vi "create_data_file.vi"(7 "Application Directory":string, 8 "Pixel":string, 9 "Device label":string, 10 "Experiment Title":string, 11 "Username":string) -> (2 "Scan number":string, 3 "Filepath out":path)   [LabVIEW 2018]
uses:
  <vilib>/Utility/file.llb/Write Delimited Spreadsheet (string).vi
panel:
  in  "device headings":string[](array[string])=["wavlength (nm)", "current (mA)", "eqe (%)"]
  in  "ref headings":string[](array[string])=["wavelength (nm)", "current (mA)"]
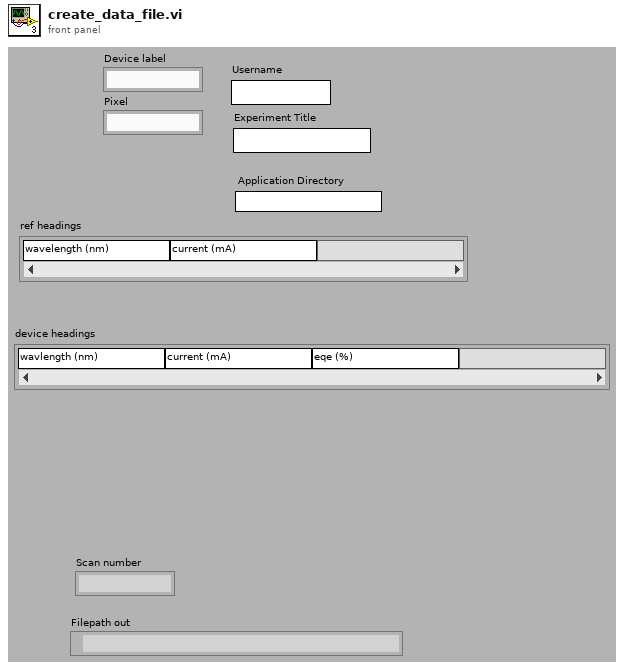
[diagram p1: front panel]
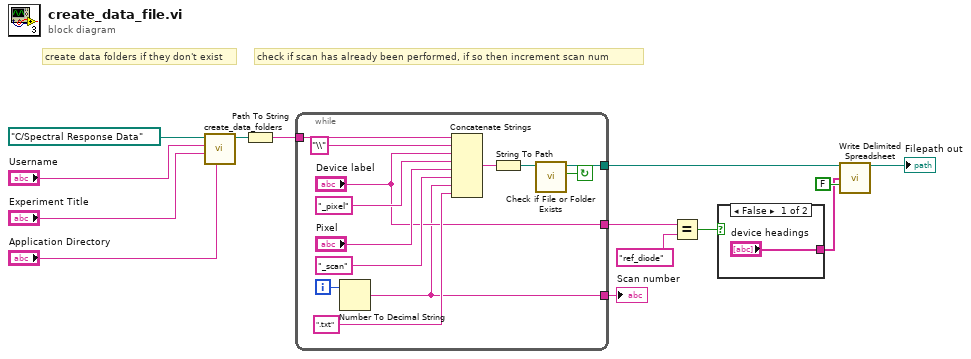
[diagram p0: block diagram]
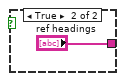
[diagram p2: hidden frame]
diagram:
  # "create data folders if they don't exist"
  # "check if scan has already been performed, if so then increment scan num"
  n1 = call "create_data_folders.vi"("Application Directory"="Application Directory", "Experiment Title"="Experiment Title", "Username"="Username", "Folderpath on C:"=path "C:/Spectral Response Data") -> ("Folderpath on C: out"=w13:path)  [unwired: 7 in]
  n2 = Path To String(path=w13) -> (string=w12:string)
  n3 = while {
    tunnel: [w18] -> w14
    tunnel: w12 -> [w27]
    tunnel: ["Device label"] -> w5
    tunnel: [w15] -> w2
    i -> [w22]
    stop <- w17 continue-if-true
    n4 = Number To Decimal String(number=w22) -> (decimal integer string=w15:string)  [unwired: 1 in]
    n5 = Concatenate Strings(w27, "\\", "Device label", "_pixel", "Pixel", "_scan", w15, ".txt" ("string")) -> (w26:string)
    n6 = String To Path(string=w26) -> (path=w19:path)
    n7 = call <vilib>:"Check if File or Folder Exists.vi"("path"=w19) -> ("file or folder exists?"=w17:bool, "dup path"=w18:path)  [unwired: 8 in, 1 out]
  }
  "Scan number" <- w2
  n8 = Equal?(x=w5, y="ref_diode") -> (x = y?=w3:bool)
  n9 = case shown="False" w3 {
    tunnel: ["device headings" "ref headings"] -> w6
    frame False {
    }
    frame True {
    }
  }
  n10 = call-poly <vilib>:"Write Delimited Spreadsheet.vi"("file path (dialog if empty)"=w14, "1D data"=w6, "append to file? (new file:F)"=FALSE) -> ("new file path (Not A Path if cancelled)"=→"Filepath out":path)  [unwired: 11 in, 1 out]
